vi "Update GraphChart LegendSD.vi"(6 "Legend:Autosize":bool, 7 "Display Type":enum16{"Chart", "Graph"}(ring), 8 "error in (no error)":errorcluster, 10 "Plot Names":string[](array[string]), 11 "GraphChart Reference in":refnum<vi>) -> (0 "error out":errorcluster, 2 "# Plots":i32, 3 "GraphChart Reference out":refnum<vi>)   [LabVIEW 2015]
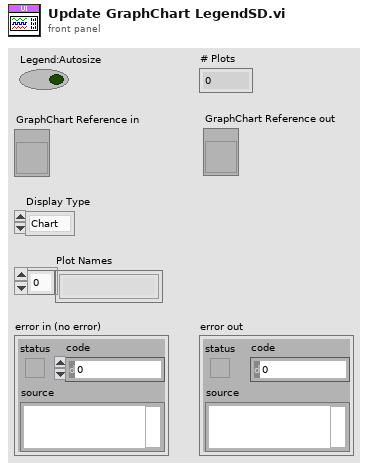
[diagram p1: front panel]
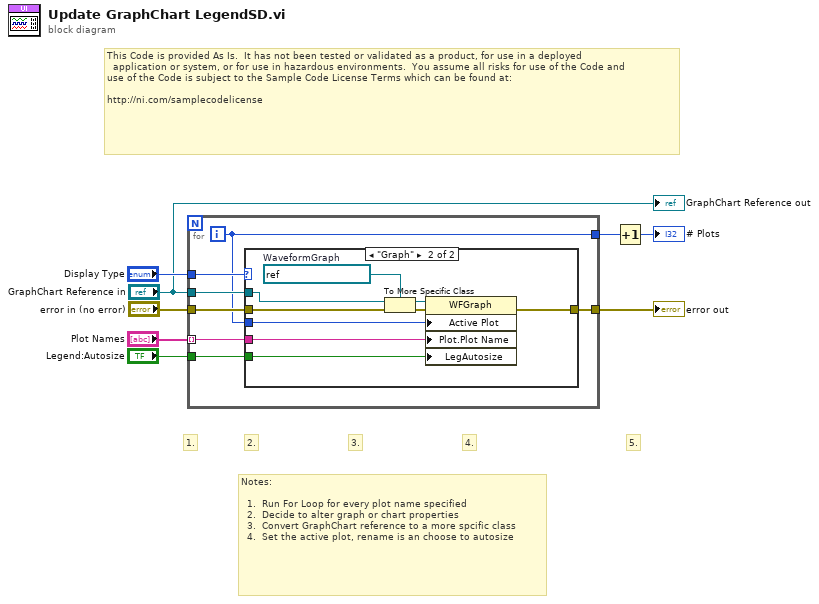
[diagram p0: block diagram]
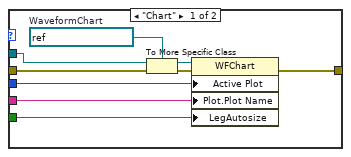
[diagram p2: hidden frame]
diagram:
  # "5."
  # "This Code is provided As Is.  It has not been tested or validated as a product, for use in a deployed\n  application or system, or for use in hazardous environments.  You assume all risks for use of the Code and   \nuse of the Code is subject to the Sample Code License Terms which can be found at: \n\nhttp://ni.com/samplecodelicense"
  # "Notes:  \n\n  1.  Run For Loop for every plot name specified  \n  2.  Decide to alter graph or chart properties\n  3.  Convert GraphChart reference to a more spcific class  \n  4.  Set the active plot, rename is an choose to autosize"
  # "4."
  # "3."
  # "2."
  # "1."
  n1 = for {
    tunnel: "Plot Names" -> [w11] mode=indexing
    tunnel: [w12] -> w3
    tunnel: "Legend:Autosize" -> [w10]
    tunnel: "GraphChart Reference in" -> [w13]
    tunnel: "Display Type" -> [w15]
    tunnel: "error in (no error)" -> [w14]
    tunnel: [w9] -> w6
    i -> [w12]
    n2 = case shown="\"Graph\"" w15 {
      tunnel: w13 -> [w23 w32]
      tunnel: [w16 w25] -> w9
      tunnel: w12 -> [w21 w28]
      tunnel: w14 -> [w20 w29]
      tunnel: w11 -> [w18 w27]
      tunnel: w10 -> [w17 w26]
      frame "Chart" {
        w24 = refnum<vi> refnum  # WaveformChart
        n3 = To More Specific Class(target class=w24, reference=w23, error in=w20) -> (specific class reference=w22:refnum<vi>, error out=w19:errorcluster)
        n4 = property class="WFChart"(reference=w22, error in=w19, "Active Plot"=w21, "Plot.Plot Name"=w18, "LegAutosize"=w17) -> (error out=w16:errorcluster)  [unwired: 1 out]
      }
      frame "Graph" {
        w33 = refnum<vi> refnum  # WaveformGraph
        n5 = To More Specific Class(target class=w33, reference=w32, error in=w29) -> (specific class reference=w31:refnum<vi>, error out=w30:errorcluster)
        n6 = property class="WFGraph"(reference=w31, error in=w30, "Active Plot"=w28, "Plot.Plot Name"=w27, "LegAutosize"=w26) -> (error out=w25:errorcluster)  [unwired: 1 out]
      }
    }
  }
  "error out" <- w6
  n7 = Increment(x=w3) -> (x+1=→"# Plots":i32)
  "GraphChart Reference out" <- "GraphChart Reference in"
